vi "Discover.vi"(0 "default reply port":u16=61558, 1 "default broadcast port":u16=61557, 5 "discovery time (ms)":u16=5000, 11 "error in (no error)":errorcluster) -> (4 "Discovered":string[](array[string]), 15 "error out":errorcluster)   [LabVIEW 2017, in "vsws.lvlib"]
uses:
  vsws.lvlib
  <vilib>/Utility/tcp.llb/UDP Multicast Write-Only Open.vi
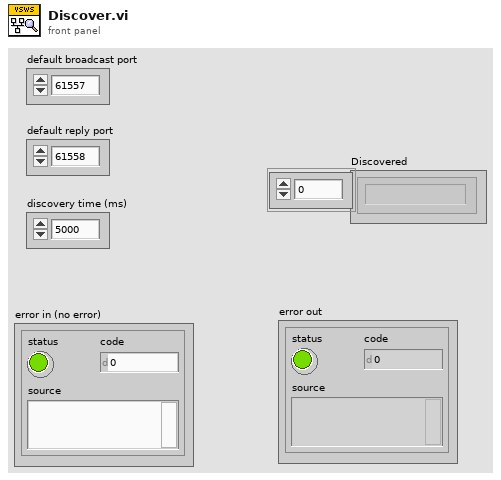
[diagram p1: front panel]
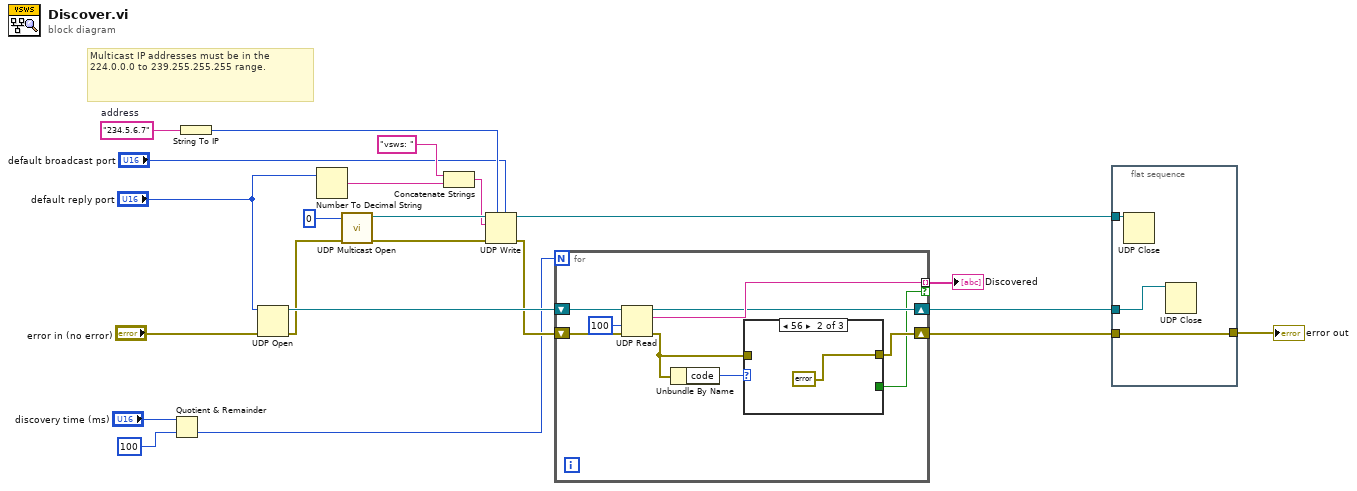
[diagram p0: block diagram]
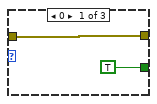
[diagram p2: hidden frame]
diagram:
  w20 = "234.5.6.7"  # address
  # "Multicast IP addresses must be in the 224.0.0.0 to 239.255.255.255 range."
  n1 = Quotient & Remainder(x="discovery time (ms)", y=u16 100) -> (floor(x/y)=w5:u16)  [unwired: 1 out]
  n2 = String To IP(1:w20) -> (0:w19:u32)
  n3 = UDP Open(8:"error in (no error)", 11:"default reply port") -> (port=w17:refnum<k16>, 0:w15:errorcluster)  [unwired: 3 in, 1 out]
  n4 = Number To Decimal String(number="default reply port") -> (decimal integer string=w12:string)  [unwired: 1 in]
  n5 = call-poly <vilib>:"UDP Multicast Open.vi"("error in (no error)"=w15, "port"=u16 0) -> ("error out"=w21:errorcluster, "connection ID"=w22:refnum<k16>)  [unwired: 8 in]
  n6 = Concatenate Strings("vsws: " ("data in"), w12) -> (w11:string)
  n7 = UDP Write(address=w19, port or service name="default broadcast port", connection ID=w22, data in=w11, 8:w21) -> (error out=w16:errorcluster, 3:w18:refnum<k16>)  [unwired: 1 in]
  n8 = for {
    N: w5 -> [_]
    tunnel: [w29] -> w4 mode=indexing if=w23
    shift-right: [w28] -> w9
    shift-left: w17 -> [w31]
    shift-right: [w24] -> w3
    shift-left: w16 -> [w30]
    n9 = UDP Read(connection ID=w31, timeout ms (25000)=100, 8:w30) -> (data out=w29:string, error out=w25:errorcluster, 3:w28:refnum<k16>)  [unwired: 1 in, 2 out]
    n10 = Unbundle By Name(w25) -> ("code"=w26:i32)
    n11 = case shown="56" w26 {
      tunnel: w25 -> [w33 _ w35]
      tunnel: [w33 errorcluster {"status"=FALSE, "code"=0, "source"=""} ("error out") w35] -> w24
      tunnel: [TRUE _ _] -> w23
      frame 0 {
      }
      frame 56 {
      }
      frame Default {
      }
    }
  }
  "Discovered" <- w4
  n12 = flat-sequence {
    tunnel: w18 -> [w38]
    tunnel: w9 -> [w37]
    tunnel: w3 -> [w36]
    tunnel: [w36] -> w2
    frame #0 {
      n13 = UDP Close(connection ID=w38) -> ()  [unwired: 1 in, 2 out]
      n14 = UDP Close(connection ID=w37) -> ()  [unwired: 1 in, 2 out]
    }
  }
  "error out" <- w2
